vi "校准数据选择表.vi"(9 "历史数据导入":T1(ring), 10 "量程下拉列表":enum16{"低量程", "高量程"}(ring), 11 "table":string="CODMn") -> (2 "布尔":bool=TRUE, 3 "输出":T2)   [LabVIEW 2016]
uses:
  <vilib>/Utility/miscctls.llb/LVPointTypeDef.ctl
  <vilib>/Utility/miscctls.llb/LVRowAndColumnUnsignedTypeDef.ctl
panel:
  in  "显示所有数据":bool caption="显示所有数据："
  in  "确定":bool
  in  "返回":bool
  in  "多列列表框":i32(listbox)
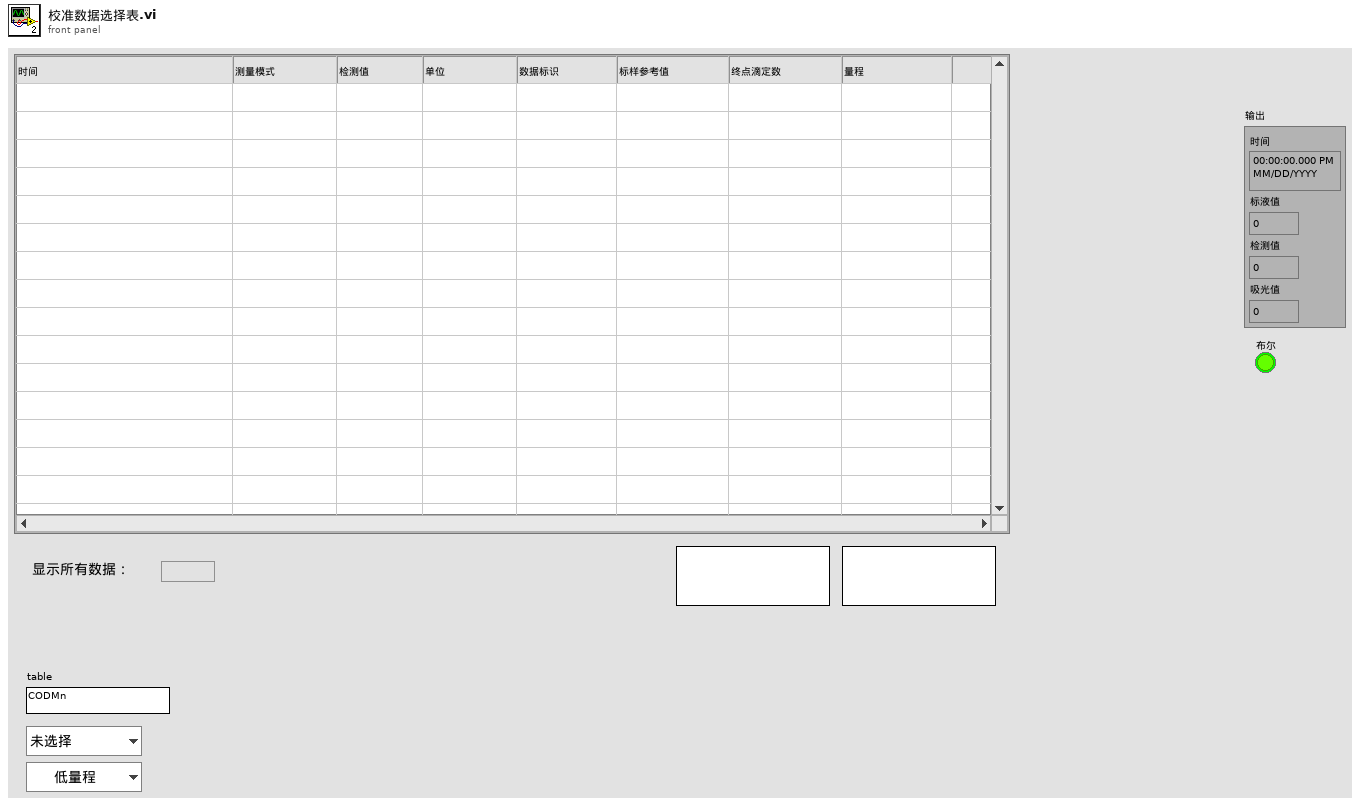
[diagram p1: front panel]
types:
  T1 = enum16{"未选择", "空白校准", "标样校准", "标样核查", "零点核查", "跨度核查"}
  T2 = cluster{"时间":timestamp, "标液值":dbl, "检测值":dbl, "吸光值":dbl}
  T3 = typedef "LVRowAndColumnUnsignedTypeDef.ctl" = cluster{"Row":u32, "Column":u32}
  T4 = typedef "LVPointTypeDef.ctl" = cluster{"Horizontal":i16, "Vertical":i16}
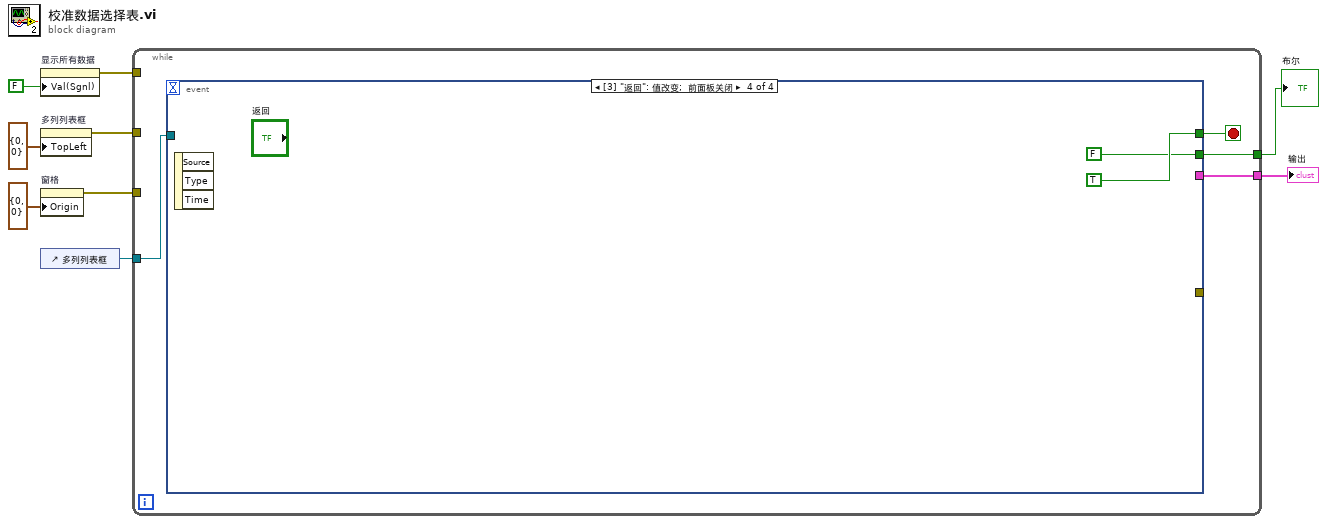
[diagram p0: block diagram]
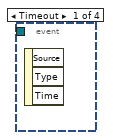
[diagram p2: hidden frame]
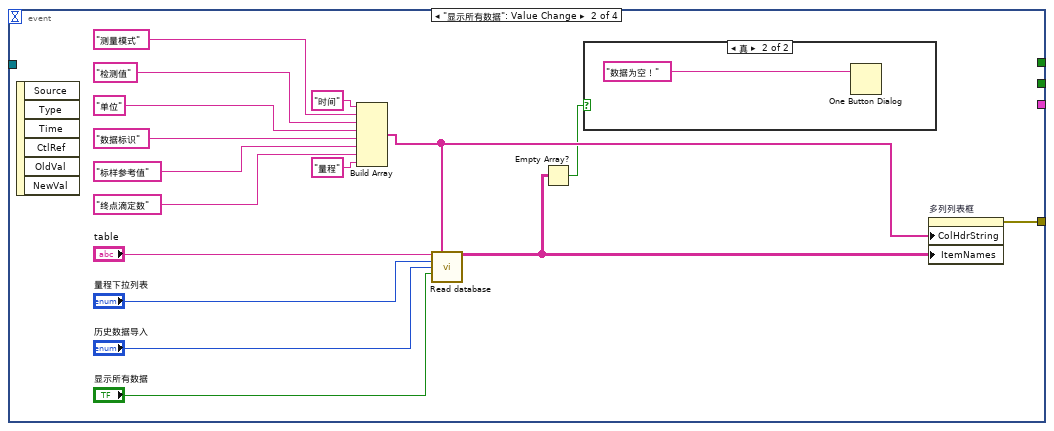
[diagram p3: hidden frame]
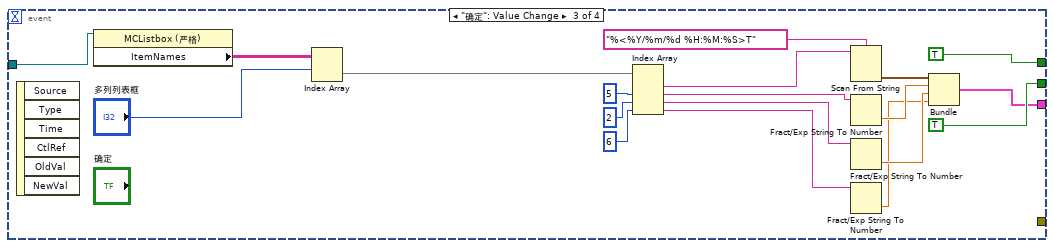
[diagram p5: hidden frame]
diagram:
  n1 = property on="显示所有数据" class="Bool (严格)"("Val(Sgnl)"=FALSE ("值(信号)")) -> (error out=w1:errorcluster)  [unwired: 2 in, 1 out]
  n2 = property on="多列列表框" class="MCListbox (严格)"("TopLeft"=T3 {"Row"=0, "Column"=0} ("左上可见单元格")) -> (error out=w3:errorcluster)  [unwired: 2 in, 1 out]
  n3 = property on="窗格" class="Pane"("Origin"=T4 {"Horizontal"=0, "Vertical"=0} ("原点")) -> (error out=w8:errorcluster)  [unwired: 2 in, 1 out]
  n4 = control-ref of="多列列表框"() -> (w5:refnum<vi>)
  n5 = while {
    tunnel: w5 -> [w12]
    tunnel: w8 -> [_]
    tunnel: [w11] -> w7
    tunnel: [w10] -> w6
    tunnel: w3 -> [_]
    tunnel: w1 -> [_]
    stop <- w13 stop-if-true
    n6 = event shown="[3] \"返回\": 值改变;  前面板关闭" {
      selector: _ -> [_ _ _ _]
      dyn-events: _ -> [_ _ _ _]
      timeout: _ -> [_ _ _ _]
      tunnel: [_ _ TRUE TRUE] -> w13
      tunnel: w12 -> [_ _ w47 _]
      tunnel: [_ _ TRUE FALSE] -> w11
      tunnel: [_ _ w34 _] -> w10
      tunnel: [_ w15 _ _] -> _
      event Timeout {
        n7 = event-data() -> ()  [unwired: 1 in, 3 out]
      }
      event "显示所有数据": Value Change {
        n8 = event-data() -> ()  [unwired: 1 in, 6 out]
        n9 = Build Array("时间", "测量模式", "检测值", "单位", "数据标识", "标样参考值", "终点滴定数", "量程") -> (w24:string[])
        n10 = call "Read database.vi"("table"="table", "显示项"=w24, "量程下拉列表"="量程下拉列表", "历史数据导入"="历史数据导入", "显示所有数据"="显示所有数据") -> ("表格"=w16:string[][])  [unwired: 7 in, 3 out]
        n11 = Empty Array?(array=w16) -> (empty?=w17:bool)
        n12 = case shown="真" w17 {
          frame False {
          }
          frame True {
            n13 = One Button Dialog(message="数据为空！" ("消息")) -> ()  [unwired: 1 in, 1 out]
          }
        }
        n14 = property on="多列列表框" class="MCListbox (严格)"("ColHdrString"=w24, "ItemNames"=w16) -> (error out=w15:errorcluster)  [unwired: 2 in, 1 out]
      }
      event "确定": Value Change {
        n15 = event-data() -> ()  [unwired: 1 in, 6 out]
        n16 = property class="MCListbox (严格)"(reference=w47) -> ("ItemNames"=w48:string[][])  [unwired: 1 in, 2 out]
        n17 = Index Array(array=w48, index (row)="多列列表框") -> (element=w44:string[])  [unwired: 1 in]
        n18 = Index Array(array=w44, index #2=5 ("索引"), index #3=2 ("索引"), index #4=6 ("索引")) -> (element #1=w32:string, element #2=w40:string, element #3=w39:string, element #4=w38:string)  [unwired: 1 in]
        n19 = Scan From String(format string="%<%Y/%m/%d %H:%M:%S>T" ("格式字符串"), input string=w32) -> (output 1=w31:timestamp)  [unwired: 3 in, 3 out]
        n20 = Fract/Exp String To Number(string=w40) -> (number=w37:dbl)  [unwired: 3 in, 1 out]
        n21 = Fract/Exp String To Number(string=w39) -> (number=w36:dbl)  [unwired: 3 in, 1 out]
        n22 = Fract/Exp String To Number(string=w38) -> (number=w35:dbl)  [unwired: 3 in, 1 out]
        n23 = Bundle(w31, w37, w36, w35) -> (w34:cluster{timestamp, dbl, dbl, dbl})  [unwired: 1 in]
      }
      event "返回": Value Change; Panel Close {
        n24 = event-data() -> ()  [unwired: 1 in, 3 out]
      }
    }
  }
  "布尔" <- w7
  "输出" <- w6
